vi "Create Message Queue.vi"(8 "에러 입력(에러 없음)":errorcluster) -> (0 "에러 출력":errorcluster, 3 "큐 출력":refnum<queue>)   [LabVIEW 2020]
uses:
  Controls/Message Cluster.ctl
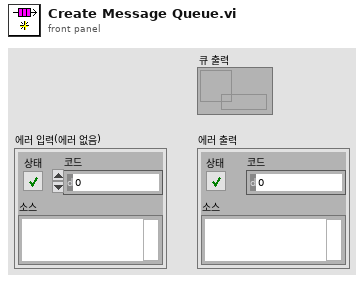
[diagram p1: front panel]
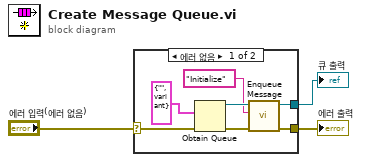
[diagram p0: block diagram]
diagram:
  n1 = case shown="에러 없음" "에러 입력(에러 없음)" {
    selector: "에러 입력(에러 없음)" -> [w9 w11]
    tunnel: [w5 _] -> w3
    tunnel: [w7 w11] -> w2
    frame No Error {
      n2 = Obtain Queue(element data type=cluster{"메세지":string, "값":variant} {"메세지"="", "값"=variant} ("Message Cluster"), error in (no error)=w9) -> (queue out=w6:refnum<queue>, error out=w8:errorcluster)  [unwired: 3 in, 1 out]
      n3 = call "Enqueue Message.vi"("에러 입력(에러 없음)"=w8, "메세지"="Initialize", "큐 입력"=w6) -> ("에러 출력"=w7:errorcluster, "큐 출력"=w5:refnum<queue>)  [unwired: 7 in]
    }
    frame Error {
    }
  }
  "큐 출력" <- w3
  "에러 출력" <- w2
